vi "DATA.vi"() -> ()   [LabVIEW 2016]
panel:
  out "IV":dbl[][](graph)=[[172.002], [172.014], [172.02], [172.032], [172.05], [172.038], [171.99], [171.984], [172.008], [172.02], [172.038], [172.032], [172.008], [171.99], [171.984], [171.99], [172.008], [172.02], [172.032], [171.996], [172.002], [172.014], [172.032], [172.056], [172.056], [172.038], [172.008], [171.996], [172.014], [172.026], [172.032], [172.044], [172.008], [171.996], [171.99], [172.014], [172.032], [172.038], [172.032], [171.99], [171.984], [171.996], [172.014], [172.032], [172.026], [172.002], [171.99], [171.996], [172.02], [172.038], [172.05], [172.032], [172.002], [172.008], [172.014], [172.032], [172.044], [172.056], [172.044], [172.002], [171.996], [172.002], [172.026], [172.038], [172.044], [172.05], [172.02], [172.002], [171.99], [172.002], [172.008], [172.026], [172.02], [171.978], [171.978], [171.984], [171.99], [171.99], [172.002], [171.978], [171.96], [171.972], [171.984], [171.99], [171.996], [171.996], [171.978], [171.954], [171.948], [171.972], [171.99], [172.008], [172.032], [172.014], [171.996], [172.008], [172.014], [172.014], [172.008], [171.99], [171.972], [171.972], [171.99], [172.008], [172.032], [172.02], [171.996], [171.984], [171.996], [172.014], [172.02], [172.002], [171.972], [171.978], [171.99], [172.008], [172.026], [172.026], [171.99], [171.978], [171.99], [171.996], [172.002], [172.002], [172.002]]
  out "IV 2":dbl[][](graph)=[[172.002], [172.014], [172.02], [172.032], [172.05], [172.038], [171.99], [171.984], [172.008], [172.02], [172.038], [172.032], [172.008], [171.99], [171.984], [171.99], [172.008], [172.02], [172.032], [171.996], [172.002], [172.014], [172.032], [172.056], [172.056], [172.038], [172.008], [171.996], [172.014], [172.026], [172.032], [172.044], [172.008], [171.996], [171.99], [172.014], [172.032], [172.038], [172.032], [171.99], [171.984], [171.996], [172.014], [172.032], [172.026], [172.002], [171.99], [171.996], [172.02], [172.038], [172.05], [172.032], [172.002], [172.008], [172.014], [172.032], [172.044], [172.056], [172.044], [172.002], [171.996], [172.002], [172.026], [172.038], [172.044], [172.05], [172.02], [172.002], [171.99], [172.002], [172.008], [172.026], [172.02], [171.978], [171.978], [171.984], [171.99], [171.99], [172.002], [171.978], [171.96], [171.972], [171.984], [171.99], [171.996], [171.996], [171.978], [171.954], [171.948], [171.972], [171.99], [172.008], [172.032], [172.014], [171.996], [172.008], [172.014], [172.014], [172.008], [171.99], [171.972], [171.972], [171.99], [172.008], [172.032], [172.02], [171.996], [171.984], [171.996], [172.014], [172.02], [172.002], [171.972], [171.978], [171.99], [172.008], [172.026], [172.026], [171.99], [171.978], [171.99], [171.996], [172.002], [172.002], [172.002]]
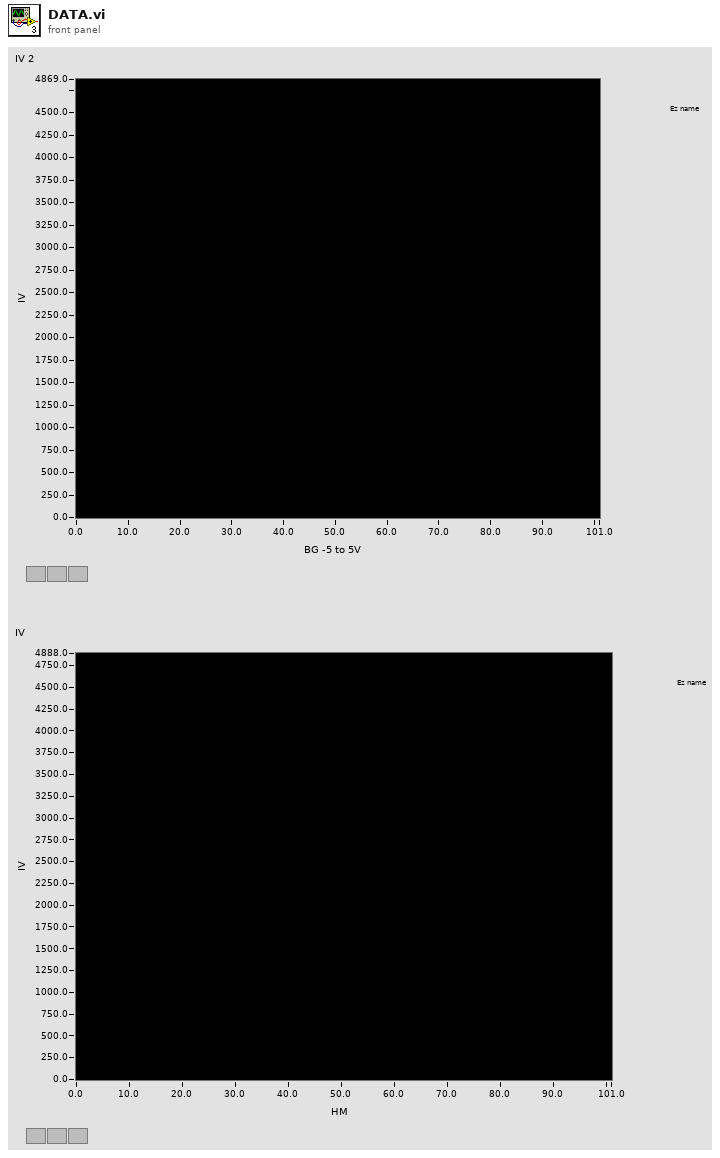
[diagram p1: front panel]
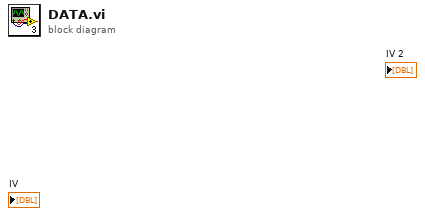
[diagram p0: block diagram]
diagram:
